vi "Create.vi"(8 "error in (no error)":errorcluster, 11 "type code":T1) -> (0 "error out":errorcluster, 3 "Type Definition out":refnum<class "Type Definition.lvclass">)   [LabVIEW 2020, in "PV Access.lvlib" / "PV Data.lvlib" / "Type Definition.lvclass"]
uses:
  Type Definition.lvclass
  Type Code.ctl
  PV Access.lvlib
  PV Data.lvlib
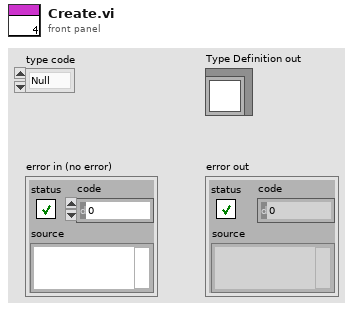
[diagram p1: front panel]
types:
  T1 = typedef "PV Access.lvlib/PV Data.lvlib/Type Code.ctl" = enum8{"Null", "Bool", "BoolA", "Int8", "Int8A", "Int16", "Int16A", "Int32", "Int32A", "Int64", "Int64A", "UInt8", "UInt8A", "UInt16", "UInt16A", "UInt32", "UInt32A", "UInt64", "UInt64A", "Float32", "Float32A", "Float64", "Float64A", "String", "StringA", "Struct", "StructA", "Union", "UnionA", "Any", "AnyA"}
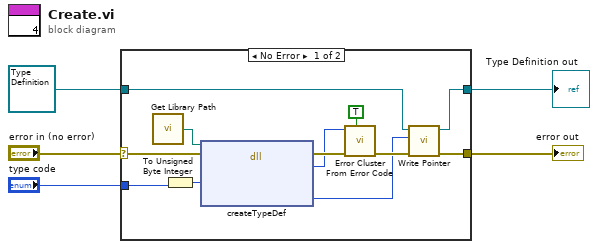
[diagram p0: block diagram]
diagram:
  n1 = case shown="No Error" "error in (no error)" {
    selector: "error in (no error)" -> [w17 w19]
    tunnel: [w10 w19] -> w3
    tunnel: refnum<class "Type Definition.lvclass"> refnum ("Type Definition in") -> [w12 w18]
    tunnel: [w11 w18] -> w2
    tunnel: "type code" -> [w7 _]
    frame No Error {
      n2 = call "Get Library Path.vi"() -> ("Path"=w13:path)  [unwired: 1 in]
      n3 = To Unsigned Byte Integer(number=w7) -> (unsigned 8bit integer=w6:u8)
      n4 = dll-call lib="?" fn="createTypeDef" ("createNT Scalar")(path in=w13, error in=w17, "type code"=w6) -> (error out=w15:errorcluster, "err_code"=w14:i32, "def"=w8:i64)  [unwired: 3 in, 1 out]
      n5 = call <vilib>:"Error Cluster From Error Code.vi"("show call chain? (False)"=TRUE, "error in (no error)"=w15, "error code (0)"=w14) -> ("error out"=w9:errorcluster)  [unwired: 6 in]
      n6 = call-dynamic "Write Pointer.vi"("error in (no error)"=w9, "Pointer"=w8, "Pointer Base in"=w12) -> ("error out"=w10:errorcluster, "Pointer Base out"=w11:refnum<class "Type Definition.lvclass">)  [unwired: 7 in]
    }
    frame Error {
    }
  }
  "error out" <- w3
  "Type Definition out" <- w2
